vi "Set or Get ActiveCell Justify.vi"(6 "Active Cell":T1 caption="活动单元格:活动单元格", 8 "error in (no error)":errorcluster caption="错误输入（无错误）", 9 "Mode":T2, 10 "Justify In":enum16{"Left", "Center", "Right"}(ring), 11 "Table Ref In":refnum<vi>) -> (0 "error out":errorcluster caption="错误输出", 2 "Justify Out":enum16{"Left", "Center", "Right"}(ring), 3 "Table Ref Out":refnum<vi>)   [LabVIEW 2013, in "Table Tool.lvlib"]
uses:
  Table Tool.lvlib
  Custum Type/GetOrSet.ctl
  <vilib>/Utility/miscctls.llb/LVRowAndColumnTypeDef.ctl
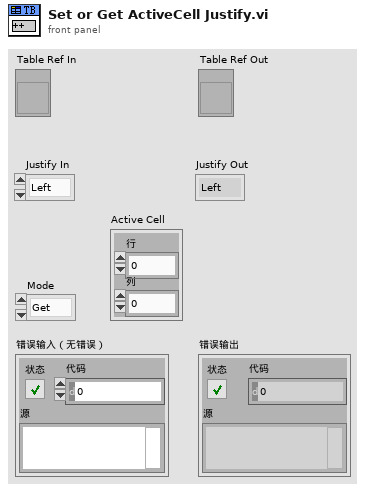
[diagram p1: front panel]
types:
  T1 = typedef "LVRowAndColumnTypeDef.ctl" = cluster{"Row":i32, "Column":i32}
  T2 = typedef "Table Tool.lvlib/GetOrSet.ctl" = enum16{"Get", "Set"}
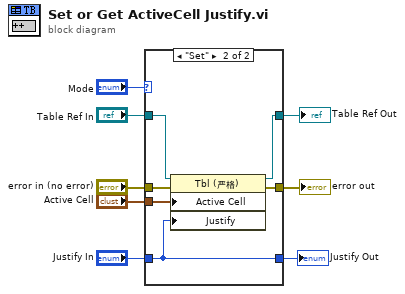
[diagram p0: block diagram]
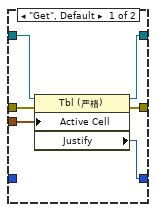
[diagram p2: hidden frame]
diagram:
  n1 = case shown="\"Set\"" "Mode" {
    tunnel: "Table Ref In" -> [w14 w19]
    tunnel: "error in (no error)" -> [w13 w20]
    tunnel: [w12 w17] -> w5
    tunnel: [w11 w18] -> w4
    tunnel: "Justify In" -> [_ w15]
    tunnel: [w10 w15] -> w2
    tunnel: "Active Cell" -> [w9 w16]
    frame "Get", Default {
      n2 = property class="Tbl (严格)"(reference=w14, error in=w13, "Active Cell"=w9) -> (reference out=w11:refnum<vi>, error out=w12:errorcluster, "Justify"=w10:enum16{"Left", "Center", "Right"})
    }
    frame "Set" {
      n3 = property class="Tbl (严格)"(reference=w19, error in=w20, "Active Cell"=w16, "Justify"=w15) -> (reference out=w18:refnum<vi>, error out=w17:errorcluster)
    }
  }
  "Table Ref Out" <- w4
  "error out" <- w5
  "Justify Out" <- w2
